vi "Configure Sysdef.vi"(4 "Target IP":string, 6 "Target Rate":dbl=1000.0, 8 "error in (no error)":errorcluster, 9 "Set DAQ timing to sample complete?":T1, 11 "UUT Path":path) -> (0 "error out":errorcluster, 3 "UUT Path dup":path)   [LabVIEW 2020]
uses:
  Sysdef Settings.ctl
  NationalInstruments.VeriStand.SystemDefinitionAPI
panel:
  out "error":string
  out "SaveSystemDefinitionFile":bool
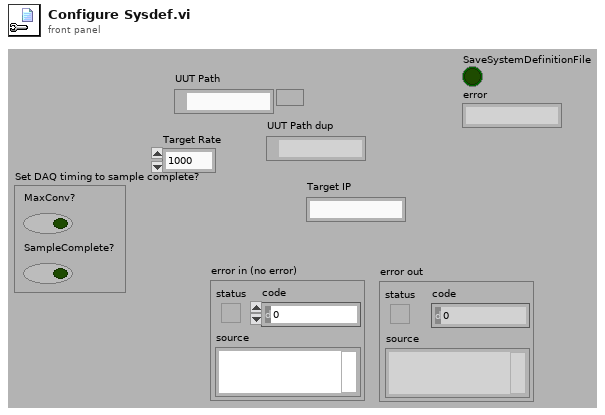
[diagram p1: front panel]
types:
  T1 = typedef "Sysdef Settings.ctl" = cluster{"MaxConv?":bool, "SampleComplete?":bool}
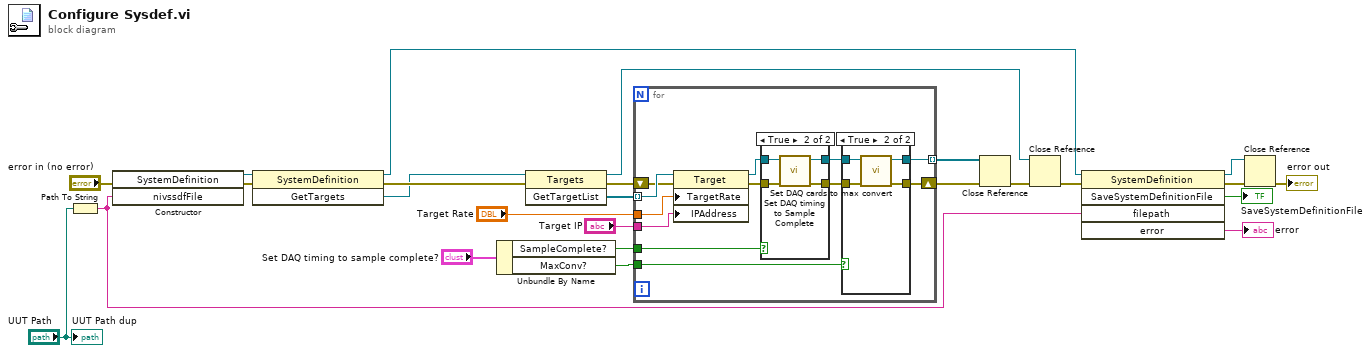
[diagram p0: block diagram]
diagram:
  n1 = Path To String(path="UUT Path") -> (string=w22:string)
  n2 = constructor class="SystemDefinition"(error in="error in (no error)", "nivssdfFile"=w22) -> (reference out=w9:refnum<k24>, error out=w8:errorcluster)  [unwired: 2 in, 2 out]
  n3 = invoke class="SystemDefinition" method="GetTargets"(reference=w9, error in=w8) -> (reference out=w7:refnum<k24>, error out=w18:errorcluster, "GetTargets"=w17:refnum<k24>)  [unwired: 1 in]
  n4 = Unbundle By Name("Set DAQ timing to sample complete?") -> ("SampleComplete?"=w11:bool, "MaxConv?"=w10:bool)
  n5 = invoke class="Targets" method="GetTargetList"(reference=w17, error in=w18) -> (reference out=w2:refnum<k24>, error out=w24:errorcluster, "GetTargetList"=w16:refnum<k24>[])  [unwired: 1 in]
  n6 = for {
    tunnel: w16 -> [w37] mode=indexing
    tunnel: [w28] -> w3 mode=indexing
    shift-right: [w27] -> w4
    shift-left: w24 -> [w36]
    tunnel: "Target Rate" -> [w35]
    tunnel: "Target IP" -> [w34]
    tunnel: w11 -> [w31]
    tunnel: w10 -> [w26]
    n7 = property class="Target"(reference=w37, error in=w36, "TargetRate"=w35, "IPAddress"=w34) -> (reference out=w32:refnum<k24>, error out=w33:errorcluster)
    n8 = case shown="True" w31 {
      tunnel: w33 -> [w45 w49]
      tunnel: w32 -> [w44 w48]
      tunnel: [w44 w47] -> w29
      tunnel: [w45 w46] -> w30
      frame False {
      }
      frame True {
        n9 = call "Set DAQ timing to Sample Complete.vi"("error in (no error)"=w49, "Target"=w48) -> ("error out"=w46:errorcluster, "Target out"=w47:refnum<k24>)  [unwired: 8 in]
      }
    }
    n10 = case shown="True" w26 {
      tunnel: w30 -> [w39 w43]
      tunnel: w29 -> [w38 w42]
      tunnel: [w38 w41] -> w28
      tunnel: [w39 w40] -> w27
      frame False {
      }
      frame True {
        n11 = call "Set DAQ cards to max convert.vi"("error in (no error)"=w43, "Target"=w42) -> ("error out"=w40:errorcluster, "Target dup"=w41:refnum<k24>)  [unwired: 8 in]
      }
    }
  }
  n12 = Close Reference(reference=w3, error in (no error)=w4) -> (error out=w5:errorcluster)
  n13 = Close Reference(reference=w2, error in (no error)=w5) -> (error out=w1:errorcluster)
  n14 = invoke class="SystemDefinition" method="SaveSystemDefinitionFile"(reference=w7, error in=w1, "filepath"=w22) -> (reference out=w25:refnum<k24>, error out=w6:errorcluster, "SaveSystemDefinitionFile"=→"SaveSystemDefinitionFile":bool, "error"=→"error":string)  [unwired: 2 in, 1 out]
  n15 = Close Reference(reference=w25, error in (no error)=w6) -> (error out=→"error out":errorcluster)
  "UUT Path dup" <- "UUT Path"
